vi "niFpgaFFTStreamingCore.vi"(0 "real data in":fxp<+/-,16,1>, 1 "reset":bool, 5 "imaginary data in":fxp<+/-,16,1>, 9 "input valid":bool=TRUE, 12 "ready for output":bool=TRUE) -> (3 "data index":u16, 4 "real data out":fxp<+/-,16,12> format="%.8g", 6 "imaginary data out":fxp<+/-,16,12> format="%.8g", 10 "output valid":bool, 14 "ready for input":bool)   [LabVIEW 2017]
uses:
  <vilib>/rvi/LocalResourceManager/LocalResourceManager.xnode
  <vilib>/rvi/FXPMathLib/basic elements/FxpDiscreteDelay/XNode/nifxpmath_DiscreteDelay.xnode
  <vilib>/rvi/DataTransferAndStorage/Container/XNode/niFpgaContainer.xnode
  <vilib>/rvi/Memory/Memory_Emulation/niFpgaMemoryEmulationRefIn.vi
  <vilib>/rvi/DataTransferAndStorage/Container/Common/niFpgaContainerGetUniqueNameForEmu.vi
  <vilib>/rvi/DataTransferAndStorage/Container/Common/niFpgaContainerSetEmuInfo.vi
  <vilib>/rvi/eio/common/nirviEmuReportErrorAndStop.vi
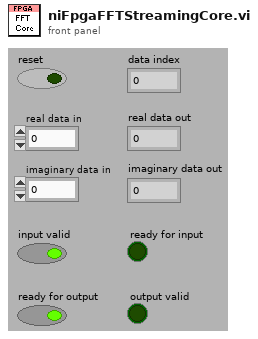
[diagram p1: front panel]
types:
  T1 = cluster{"x_r":fxp<+/-,16,1>, "x_i ":fxp<+/-,16,1>, "y_r ":fxp<+/-,16,1>, "y_i ":fxp<+/-,16,1>}
  T2 = cluster{"iteration count":u16, "lty_count":u16, "idxv":bool, "os":bool}
  T3 = cluster{"tf_count":u16, "lty_count":u16, "idxv":bool, "os":bool}
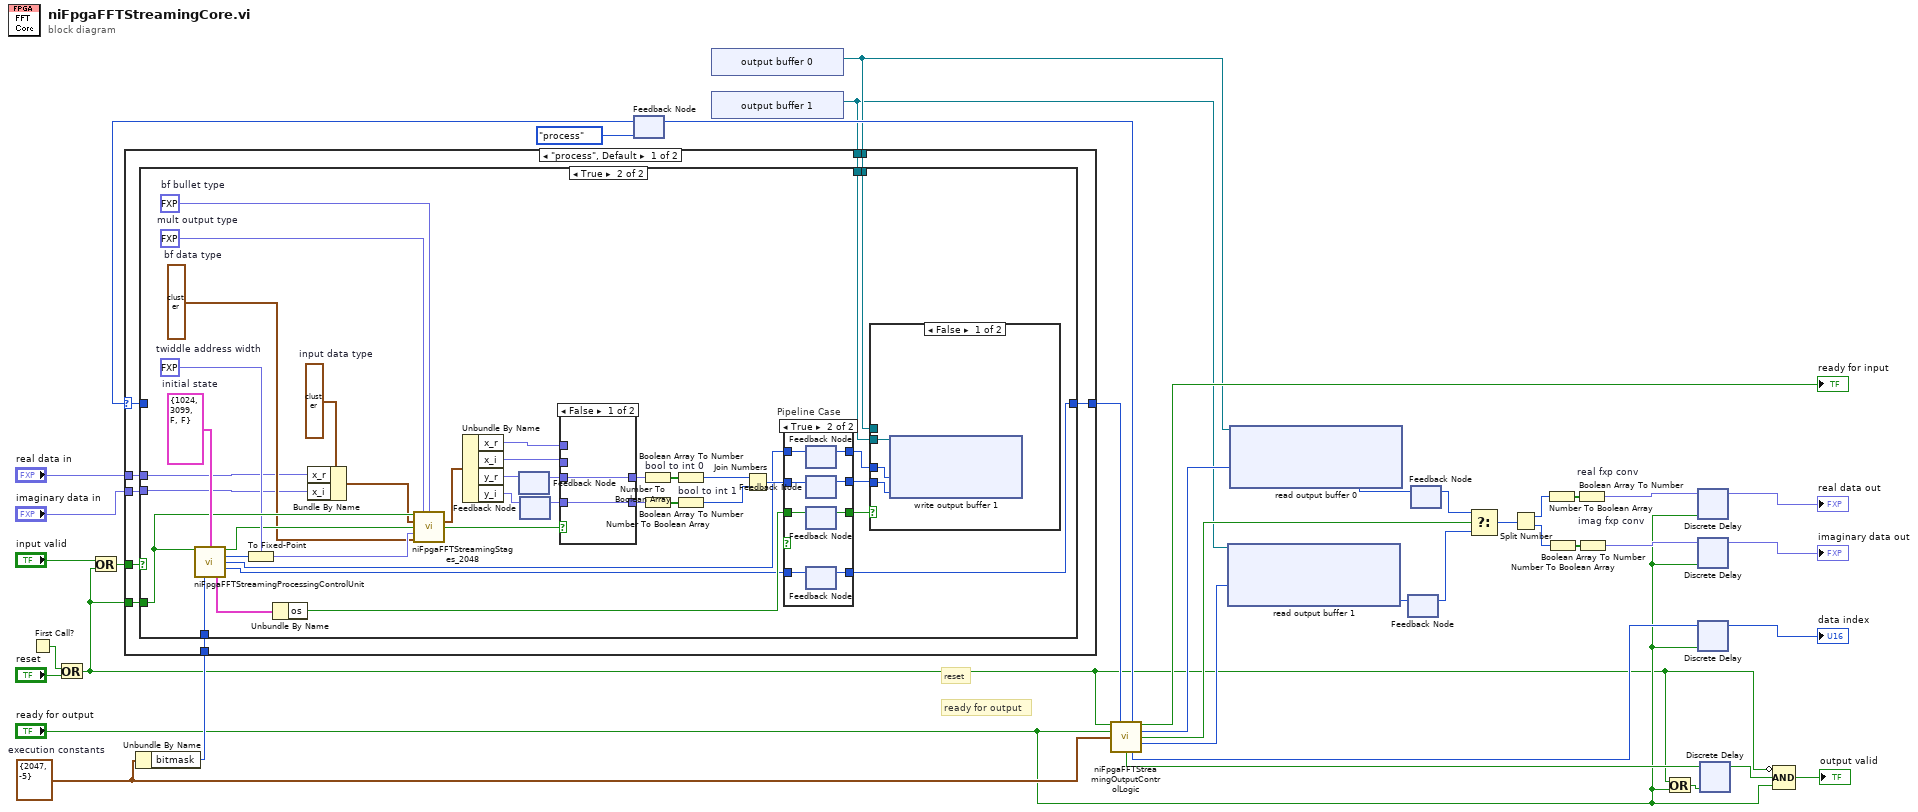
[diagram p0: block diagram]
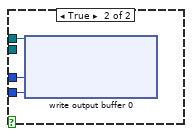
[diagram p4: hidden frame]
diagram:
  w30 = cluster{"bitmask":u16, "K-16":i8} {"bitmask"=2047, "K-16"=-5}  # execution constants
  # "reset"
  # "ready for output"
  n1 = First Call?() -> (First Call?: T/F=w6:bool)
  n2 = Or(x=w6, y="reset") -> (x .or. y?=w3:bool)
  n3 = Or(x="input valid", y=w3) -> (x .or. y?=w35:bool)
  n4 = Unbundle By Name(w30) -> ("bitmask"=w29:u16)
  n5 = feedback #1(enum8{"process", "idle"}."process") -> (w39:enum8{"process", "idle"})
  n6 = xnode "output buffer 0"() -> ("Memory Out"=w2:refnum<k21>)
  n7 = xnode "output buffer 1"() -> ("Memory Out"=w1:refnum<k21>)
  n8 = case shown="\"process\", Default" w39 {
    selector: w39 -> [w42 w111]
    tunnel: w35 -> [w48 _]
    tunnel: w3 -> [w47 _]
    tunnel: "real data in" -> [w46 _]
    tunnel: "imaginary data in" -> [w45 _]
    tunnel: [w44 w111] -> w34
    tunnel: w29 -> [w43 _]
    tunnel: w2 -> [w41 _]
    tunnel: w1 -> [w40 _]
    frame "process", Default {
      n9 = case shown="True" w48 {
        tunnel: w46 -> [_ w61]
        tunnel: w45 -> [_ w60]
        tunnel: w47 -> [_ w75]
        tunnel: [w49 w52] -> w44
        tunnel: w43 -> [_ w73]
        tunnel: w42 -> [w49 _]
        tunnel: w41 -> [_ w51]
        tunnel: w40 -> [_ w50]
        frame False {
        }
        frame True {
          w63 = T1 {"x_r"=0.0, "x_i "=0.0, "y_r "=0.0, "y_i "=0.0}  # input data type
          w65 = fxp<+/-,22,4> 0.0  # bf bullet type
          w66 = fxp<+/-,18,2> 0.0  # mult output type
          w64 = T1 {"x_r"=0.0, "x_i "=0.0, "y_r "=0.0, "y_i "=0.0}  # bf data type
          w76 = T2 {"iteration count"=1024, "lty_count"=3099, "idxv"=FALSE, "os"=FALSE}  # initial state
          w74 = fxp<+,10,10> 0.0  # twiddle address width
          n10 = call <vilib>:"niFpgaFFTStreamingProcessingControlUnit.vi"("reset"=w75, "initial state"=w76, "bitmask"=w73) -> ("stage switch"=w67:bool, "twiddle address"=w77:u16, "data index"=w55:u16, "next state"=w53:enum8{"process", "idle"}, "state out"=w78:T3)  [unwired: 4 in, 4 out]
          n11 = To Fixed-Point(fixed-point type=w74, number=w77) -> (fixed-point=w68:fxp<+,10,10>)
          n12 = Unbundle By Name(w78) -> ("os"=w57:bool)
          n13 = Bundle By Name(cluster=w63, "x_r"=w61, "x_i"=w60) -> (w62:T1)
          n14 = call <vilib>:"niFpgaFFTStreamingStages_2048.vi"("reset"=w75, "mult output type"=w66, "bf bullet type"=w65, "bf data in"=w62, "stage switch in"=w67, "twiddle index in"=w68, "bf data type"=w64) -> ("bf data out"=w70:T1, "stage switch out"=w69:bool)  [unwired: 1 in, 6 out]
          n15 = Unbundle By Name(w70) -> ("x_r"=w86:fxp<+/-,16,1>, "x_i"=w85:fxp<+/-,16,1>, "y_r"=w84:fxp<+/-,16,1>, "y_i"=w83:fxp<+/-,16,1>)
          n16 = feedback-in #2(w84) -> ()
          n17 = feedback #2() -> (w87:fxp<+/-,16,1>)  [unwired: 1 out]
          n18 = feedback-in #3(w83) -> ()
          n19 = feedback #3() -> (w88:fxp<+/-,16,1>)  [unwired: 1 out]
          n20 = case shown="False" w69 {
            tunnel: [w108 w110] -> w72
            tunnel: w85 -> [_ w110]
            tunnel: w88 -> [w108 _]
            tunnel: w87 -> [w107 _]
            tunnel: w86 -> [_ w109]
            tunnel: [w107 w109] -> w71
            frame False {
            }
            frame True {
            }
          }
          n21 = Number To Boolean Array(number=w71) -> (Boolean array=w82:bool[])
          n22 = Number To Boolean Array(number=w72) -> (Boolean array=w81:bool[])
          n23 = Boolean Array To Number "bool to int 0"(Boolean array=w82) -> (number=w80:u16)
          n24 = Boolean Array To Number "bool to int 1"(Boolean array=w81) -> (number=w79:u16)
          n25 = Join Numbers(hi=w80, lo=w79) -> ((hi.lo)=w59:u32)
          n26 = case "Pipeline Case" shown="True" {
            selector: _ -> [_ _]
            tunnel: w59 -> [w91 w100]
            tunnel: [w91 w99] -> w58
            tunnel: w57 -> [w89 w98]
            tunnel: [w89 w97] -> w56
            tunnel: w55 -> [w92 w96]
            tunnel: [w92 w95] -> w54
            tunnel: w53 -> [w90 w94]
            tunnel: [w90 w93] -> w52
            frame False {
            }
            frame True {
              n27 = feedback-in #4(w96) -> ()
              n28 = feedback #4() -> (w95:u16)  [unwired: 1 in]
              n29 = feedback-in #5(w100) -> ()
              n30 = feedback #5() -> (w99:u32)  [unwired: 1 in]
              n31 = feedback-in #6(w98) -> ()
              n32 = feedback #6() -> (w97:bool)  [unwired: 1 in]
              n33 = feedback-in #7(w94) -> ()
              n34 = feedback #7() -> (w93:enum8{"process", "idle"})  [unwired: 1 in]
            }
          }
          n35 = case shown="False" w56 {
            tunnel: w54 -> [w103 w106]
            tunnel: w58 -> [w102 w105]
            tunnel: w51 -> [_ w104]
            tunnel: w50 -> [w101 _]
            frame False {
              n36 = xnode "write output buffer 1"("Address"=w103, "Data"=w102, "Memory In"=w101) -> ()  [unwired: 1 out]
            }
            frame True {
              n37 = xnode "write output buffer 0"("Address"=w106, "Data"=w105, "Memory In"=w104) -> ()  [unwired: 1 out]
            }
          }
        }
      }
    }
    frame "idle" {
    }
  }
  n38 = call <vilib>:"niFpgaFFTStreamingOutputControlLogic.vi"("reset"=w3, "process state in"=w34, "ready for output"="ready for output", "execution constants"=w30) -> ("process state out"=w31:enum8{"process", "idle"}, "ready for input"=→"ready for input":bool, "read address 0"=w22:u16, "use buffer 0"=w18:bool, "read address 1"=w8:u16, "output valid"=w16:bool, "data index"=w14:u16)  [unwired: 5 out]
  n39 = feedback-in #1(w31) -> ()
  n40 = xnode "read output buffer 1"("Address"=w8, "Memory In"=w1) -> ("Data"=w23:u32)  [unwired: 1 out]
  n41 = xnode "read output buffer 0"("Address"=w22, "Memory In"=w2) -> ("Data"=w24:u32)  [unwired: 1 out]
  n42 = feedback-in #8(w23) -> ()
  n43 = feedback #8() -> (w19:u32)  [unwired: 1 out]
  n44 = feedback-in #9(w24) -> ()
  n45 = feedback #9() -> (w20:u32)  [unwired: 1 out]
  n46 = Select(t=w20, s=w18, f=w19) -> (s? t:f=w21:u32)
  n47 = Split Number(x=w21) -> (hi(x)=w28:u16, lo(x)=w26:u16)
  n48 = Number To Boolean Array(number=w28) -> (Boolean array=w27:bool[])
  n49 = Number To Boolean Array(number=w26) -> (Boolean array=w25:bool[])
  n50 = Boolean Array To Number "real fxp conv"(Boolean array=w27) -> (number=w12:fxp<+/-,16,12>)
  n51 = Boolean Array To Number "imag fxp conv"(Boolean array=w25) -> (number=w10:fxp<+/-,16,12>)
  n52 = Or(x=w3, y="ready for output") -> (x .or. y?=w5:bool)
  n53 = xnode ("Discrete Delay")("D"=w12, "enable"="ready for output") -> ("Q"=→"real data out":fxp<+/-,16,12>)
  n54 = xnode ("Discrete Delay")("D"=w10, "enable"="ready for output") -> ("Q"=→"imaginary data out":fxp<+/-,16,12>)
  n55 = xnode ("Discrete Delay")("D"=w14, "enable"="ready for output") -> ("Q"=→"data index":u16)
  n56 = xnode ("Discrete Delay")("D"=w16, "enable"=w5) -> ("Q"=w17:bool)
  n57 = Compound Arithmetic op=AND(invert w3, w17, "ready for output") -> (→"output valid":bool)
